vi "Rawdata_Generator.vi"() -> ()   [LabVIEW 2020]
uses:
  ctl/Image_Configuration.ctl
panel:
  in  "Files Pre fix":string
  in  "Base Imagedata Binary File":path
  in  "Post File":string="dataSource_Post_Side.txt"
  in  "Pre File":string="dataSource_Pre_Side.txt"
  in  "stop":bool
  out "Progress":dbl(slide) scale=0.0..100.0
  out "error out":errorcluster
  in  "Output File Folder":path
  in  "Timestamp Type":enum16{"Base", "Base +/- Rand(Delta T)"}(ring)=enum."Base +/- Rand(Delta T)"
  in  "Delta T (ns)":u64=1000000
  in  "Base Relative Time (ns)":u64=33000000
  in  "Num of Frames to generate":u32=5000
  in  "T0":timestamp
  in  "Image Data Type":u8=44 format="%x"
  in  "Image Configuration":T1={"Width"=1920, "Height"=1536}
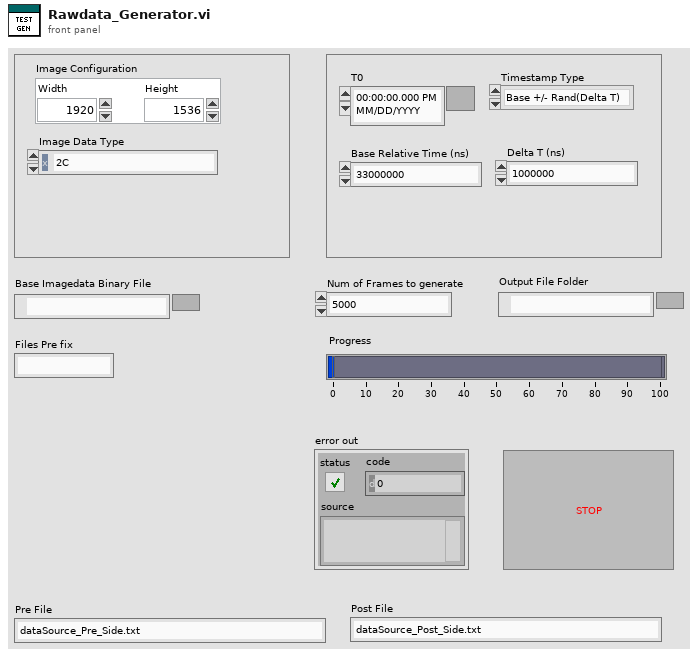
[diagram p1: front panel]
types:
  T1 = typedef "Image_Configuration.ctl" = cluster{"Width":i32, "Height":i32}
  T2 = enum16{"big-endian, network order", "native, host order", "little-endian"}
  T3 = enum16{"open", "replace", "create", "open or create", "replace or create", "replace or create with confirmation"}
  T4 = typedef "Image_Data_Config.ctl" = cluster{"Lines of Image Data":u16, "Bytes per Even Line":u16, "Bytes per Odd Line":u16, "Image Data Type":u8, "Total Image Data Block Size":u32, "Image Data Block Offset":u32}
  T5 = typedef "Image_EBD_Config.ctl" = cluster{"Lines of Pre-EBD Data":u16, "Lines of Post-EBD Data":u16, "Total EBD Block Size":u32, "Pre-EBD Block Offset ":u32, "Post-EBD Block Offset ":u32}
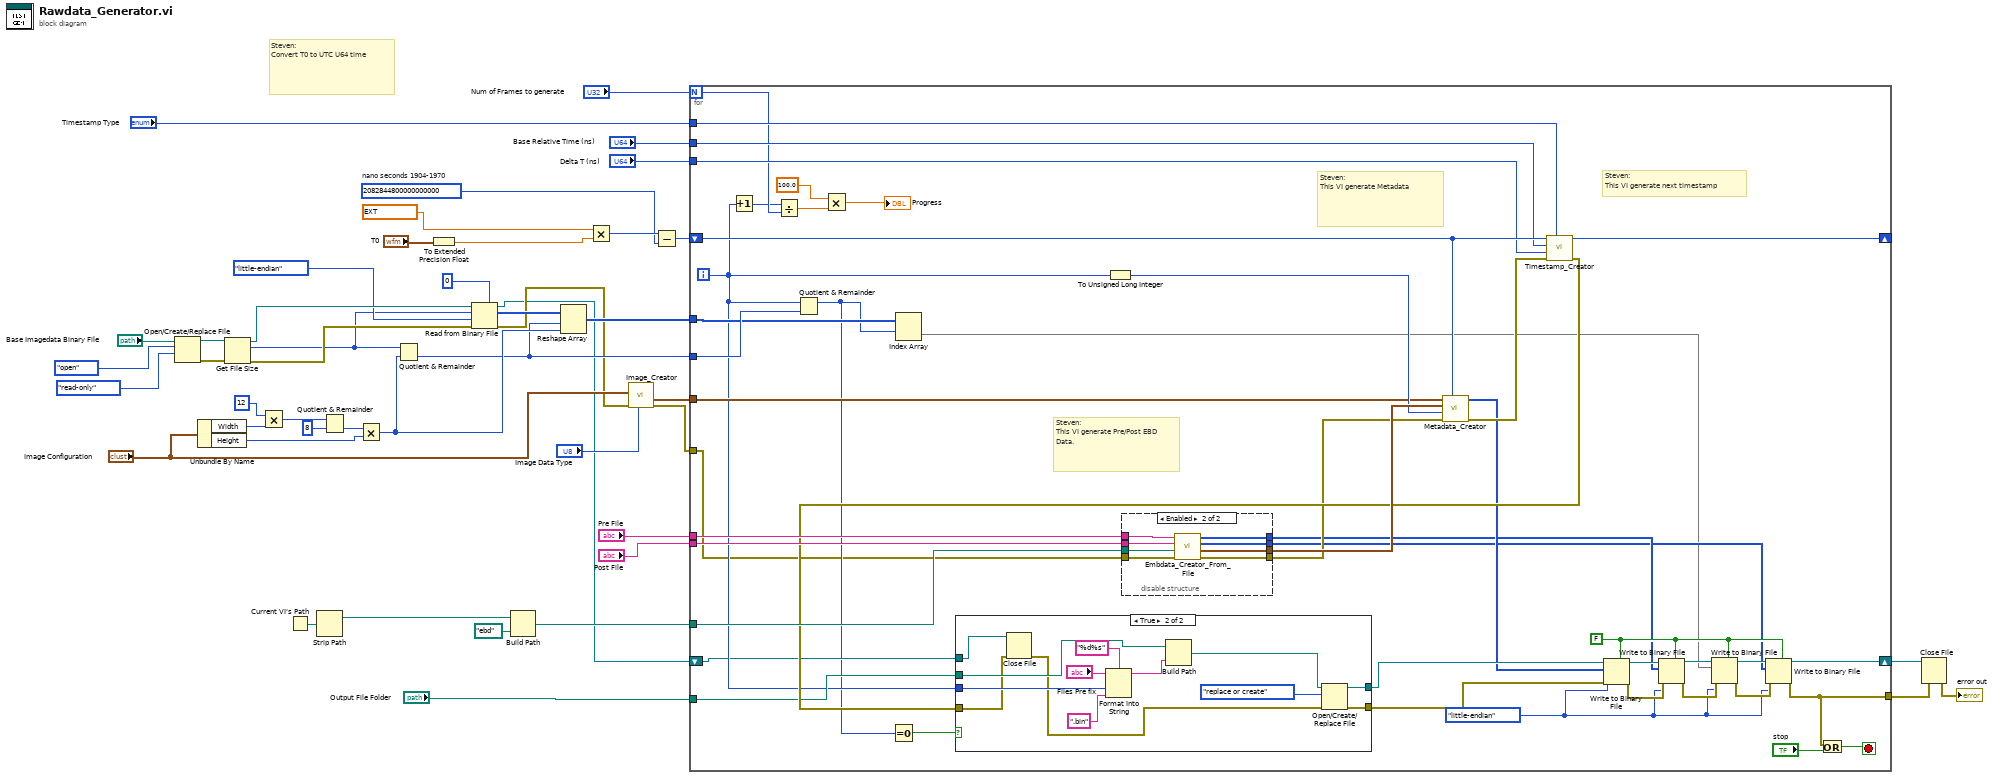
[diagram p0: block diagram]
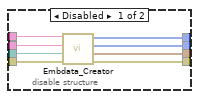
[diagram p2: hidden frame]
diagram:
  w42 = u64 2082844800000000000  # nano seconds 1904-1970
  # "Steven:\nConvert T0 to UTC U64 time"
  n1 = Open/Create/Replace File(file path (use dialog)="Base Imagedata Binary File", operation (0:open)=T3."open", access (0:read/write)=enum16{"read/write", "read-only", "write-only"}."read-only") -> (refnum out=w23:refnum<file>, error out=w24:errorcluster)  [unwired: 3 in, 1 out]
  n2 = Unbundle By Name("Image Configuration") -> ("Width"=w22:i32, "Height"=w17:i32)
  n3 = Get File Size(file=w23, error in=w24) -> (refnum out=w15:refnum<file>, size (in bytes)=w12:i64, 0:w14:errorcluster)
  n4 = Multiply(x=12, y=w22) -> (x*y=w20:i32)
  n5 = Current VI's Path() -> (path=w31:path)
  n6 = Strip Path(path=w31) -> (stripped path=w30:path)  [unwired: 1 out]
  n7 = Quotient & Remainder(x=w20, y=8) -> (floor(x/y)=w18:i32)  [unwired: 1 out]
  n8 = Multiply(x=w18, y=w17) -> (x*y=w9:i32)
  n9 = Quotient & Remainder(x=w12, y=w9) -> (floor(x/y)=w4:i64)  [unwired: 1 out]
  n10 = To Extended Precision Float(1:"T0") -> (0:w43:ext)
  n11 = Read from Binary File(5:u8 0, 8:w14, 9:T2."little-endian" ("byte order (0:big-endian, network order)"), 10:w12, 11:w15) -> (0:w2:errorcluster, 2:w10:u8[], 3:w1:refnum<file>)  [unwired: 1 in, 1 out]
  n12 = Build Path(base path=w30, name or relative path=path "ebd") -> (appended path=w28:path)
  n13 = Reshape Array(w10, w4, w9) -> (w8:u8[][])
  n14 = Multiply(x=ext 1000000000.0, y=w43) -> (x*y=w44:u64)
  n15 = call "Image_Creator.vi"("Image Data Type"="Image Data Type", "error in (no error)"=w2, "Image Configuration"="Image Configuration") -> ("error out"=w5:errorcluster, "Image Data Config"=w16:T4)  [unwired: 5 in, 2 out]
  n16 = Subtract(x=w44, y=w42) -> (x-y=w39:u64)
  n17 = for {
    N: "Num of Frames to generate" -> [w74]
    shift-right: [w84] -> _
    shift-left: w39 -> [w88]
    tunnel: "Timestamp Type" -> [w87]
    tunnel: "Base Relative Time (ns)" -> [w86]
    tunnel: "Delta T (ns)" -> [w85]
    tunnel: [w69] -> w35
    tunnel: "Pre File" -> [w67]
    tunnel: "Post File" -> [w66]
    tunnel: w28 -> [w65]
    tunnel: w16 -> [w63]
    tunnel: w8 -> [w61]
    tunnel: w5 -> [w51]
    tunnel: w4 -> [w62]
    tunnel: "Output File Folder" -> [w58]
    shift-right: [w75] -> w36
    shift-left: w1 -> [w54]
    i -> [w57]
    stop <- w68 stop-if-true
    w77 = FALSE ("prepend array or string size? (T)")
    w76 = T2."little-endian" ("byte order (0:big-endian, network order)")
    # "Steven:\nThis VI generate Metadata"
    # "Steven:\nThis VI generate Pre/Post EBD Data."
    # "Steven:\nThis VI generate next timestamp"
    n18 = Increment(x=w57) -> (x+1=w64:i32)
    n19 = Divide(x=w64, y=w74) -> (x/y=w73:dbl)
    n20 = Quotient & Remainder(x=w57, y=w62) -> (x-y*floor(x/y)=w52:i64)  [unwired: 1 out]
    n21 = Multiply(x=100.0, y=w73) -> (x*y=→"Progress":dbl)
    n22 = Equal To 0?(x=w52) -> (x = 0?=w60:bool)
    n23 = Index Array(array=w61, index (row)=w52) -> (element=w47:u8[])  [unwired: 1 in]
    n24 = To Unsigned Long Integer(number=w57) -> (unsigned 32bit integer=w90:u32)
    n25 = disable-structure shown="Enabled" {
      disable-tunnel: [w99 w101] -> w91
      disable-tunnel: w67 -> [w98 w107]
      disable-tunnel: w66 -> [w97 w106]
      disable-tunnel: w65 -> [w96 w105]
      disable-tunnel: [w95 w100] -> w53
      disable-tunnel: w51 -> [w94 w104]
      disable-tunnel: [w93 w103] -> w49
      disable-tunnel: [w92 w102] -> w48
      frame Disabled {
        n26 = call "Embdata_Creator.vi"("Pre File"=w98, "Post File"=w97, "root path"=w96, "error in (no error)"=w94) -> ("Pre-EBD Data (U8)"=w93:u8[], "Post-EBD Data (U8)"=w92:u8[], "EBD Config"=w99:T5, "error out"=w95:errorcluster)  [unwired: 3 in]
      }
      frame Enabled {
        n27 = call "Embdata_Creator_From_File.vi"("error in (no error)"=w104, "root path"=w105, "Post File"=w106, "Pre File"=w107) -> ("error out"=w100:errorcluster, "EBD Config"=w101:T5, "Post-EBD Data (U8)"=w102:u8[], "Pre-EBD Data (U8)"=w103:u8[])  [unwired: 4 in]
      }
    }
    n28 = call "Metadata_Creator.vi"("Frame Timestamp"=w88, "error in (no error)"=w53, "Frame Index"=w90, "EBD Config"=w91, "Image Data Config"=w63) -> ("error out"=w89:errorcluster, "Meta Data (U8)"=w50:u8[])  [unwired: 5 in]
    n29 = call "Timestamp_Creator.vi"("Timestamp Type"=w87, "error in (no error)"=w89, "Delta T (ns)"=w85, "Base Relative Time (ns)"=w86, "Previous Time (ns)"=w88) -> ("error out"=w59:errorcluster, "Next Time (ns)"=w84:u64)  [unwired: 5 in]
    n30 = case shown="True" w60 {
      tunnel: w59 -> [w108 w111]
      tunnel: w58 -> [_ w118]
      tunnel: w57 -> [_ w122]
      tunnel: [w109 w114] -> w55
      tunnel: [w108 w113] -> w56
      tunnel: w54 -> [w109 w112]
      frame False {
      }
      frame True {
        n31 = Close File(refnum=w112, error in=w111) -> (error out=w110:errorcluster)  [unwired: 1 out]
        n32 = Format Into String(format string="%d%s", initial string="Files Pre fix", w122, ".bin") -> (resulting string=w117:string)  [unwired: 1 in, 1 out]
        n33 = Build Path(base path=w118, name or relative path=w117) -> (appended path=w116:path)
        n34 = Open/Create/Replace File(file path (use dialog)=w116, error in=w110, operation (0:open)=T3."replace or create") -> (refnum out=w114:refnum<file>, error out=w113:errorcluster)  [unwired: 3 in, 1 out]
      }
    }
    n35 = Write to Binary File(file (use dialog)=w55, data=w50, error in=w56, 5:w77, 9:w76) -> (refnum out=w83:refnum<file>, error out=w82:errorcluster)  [unwired: 1 in, 1 out]
    n36 = Write to Binary File(file (use dialog)=w83, data=w49, error in=w82, 5:w77, 9:w76) -> (refnum out=w81:refnum<file>, error out=w80:errorcluster)  [unwired: 1 in, 1 out]
    n37 = Write to Binary File(file (use dialog)=w81, data=w47, error in=w80, 5:w77, 9:w76) -> (refnum out=w79:refnum<file>, error out=w78:errorcluster)  [unwired: 1 in, 1 out]
    n38 = Write to Binary File(file (use dialog)=w79, data=w48, error in=w78, 5:w77, 9:w76) -> (refnum out=w75:refnum<file>, error out=w69:errorcluster)  [unwired: 1 in, 1 out]
    n39 = Or(x=w69, y="stop") -> (x .or. y?=w68:bool)
  }
  n40 = Close File(refnum=w36, error in=w35) -> (error out=→"error out":errorcluster)  [unwired: 1 out]
